vi "SVT Telecommunications Weighting Filter (frequency).vi"   [LabVIEW 2017, in "SoundVib_TeleWeighting.lvlib"]
doc: "Applies the selected telecommunications weighting to a previously computed frequency spectrum or spectra. This VI weights each spectral bin according to the attenuation of the specified filter at the bin center frequency. You can use this VI in a loop to process multiple blocks. Wire data to the<B> spectrum</B> input to determine the polymorphic instance to use or manually select the instance."
uses:
  <vilib>/addons/Sound and Vibration/svt_Weighting/SoundVib_TeleWeighting.lvlib
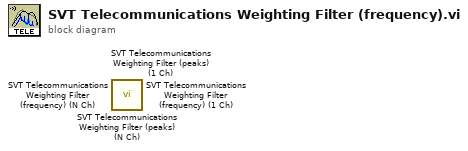
[diagram p0: block diagram]
diagram:
  n1 = call <vilib>:"SVT Telecommunications Weighting Filter (peaks) (N Ch).vi"() -> ()  [unwired: 16 in, 4 out]
  n2 = call <vilib>:"SVT Telecommunications Weighting Filter (peaks) (1 Ch).vi"() -> ()  [unwired: 16 in, 4 out]
  n3 = call <vilib>:"SVT Telecommunications Weighting Filter (frequency) (N Ch).vi"() -> ()  [unwired: 16 in, 4 out]
  n4 = call <vilib>:"SVT Telecommunications Weighting Filter (frequency) (1 Ch).vi"() -> ()  [unwired: 16 in, 4 out]
